vi "motor step1.vi"(8 "error in (no error)":errorcluster, 9 "direction":enum16{"counter-clockwise", "clockwise"}(ring), 10 "steps":i32=1, 11 "Handle In":i32) -> (0 "error out":errorcluster, 2 "steps performed":i32, 3 "Handle Out":i32)   [LabVIEW 2013]
uses:
  motor constants.ctl
  motor global state actions.ctl
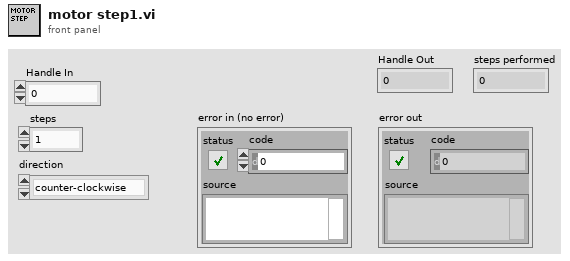
[diagram p1: front panel]
types:
  T1 = typedef "motor global state actions.ctl" = enum16{"set value", "get value", "set angle", "set initialized", "set complete", "set handle", "get handle"}
  T2 = typedef "motor constants.ctl" = u16
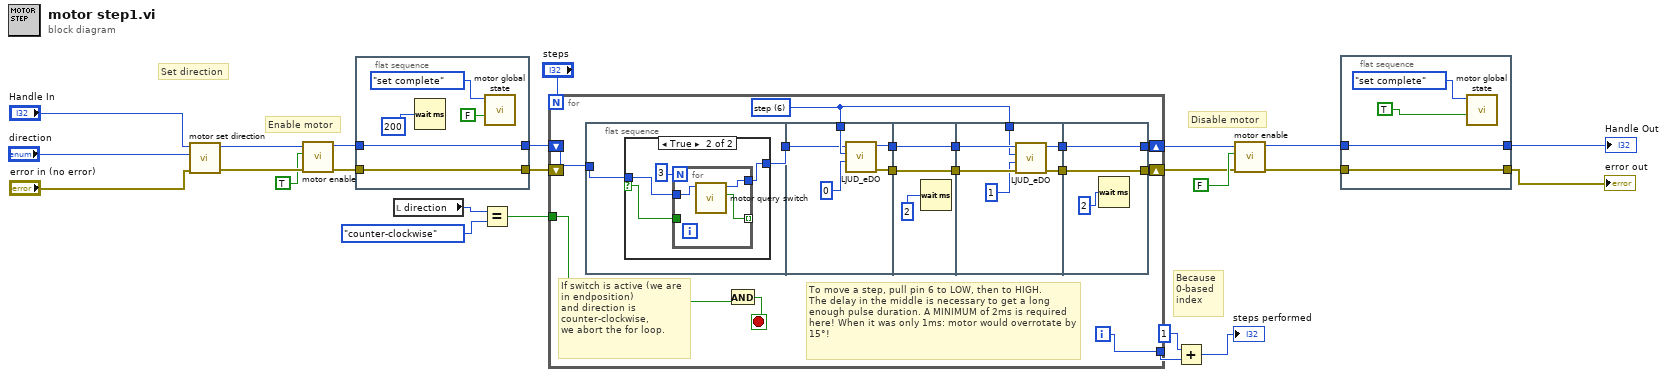
[diagram p0: block diagram]
diagram:
  # "Because \n0-based \nindex"
  # "Disable motor"
  # "Enable motor"
  # "Set direction"
  n1 = call "motor set direction.vi"("error in (no error)"="error in (no error)", "direction"="direction", "Handle In"="Handle In") -> ("error out"=w11:errorcluster, "Handle Out"=w10:i32)  [unwired: 7 in]
  n2 = call "motor enable.vi"("error in (no error)"=w11, "enable"=TRUE, "Handle In"=w10) -> ("error out"=w13:errorcluster, "Handle Out"=w12:i32)  [unwired: 7 in]
  n3 = flat-sequence {
    tunnel: w12 -> [w28]
    tunnel: w13 -> [w29]
    tunnel: [w29] -> w20
    tunnel: [w28] -> w19
    frame #0 {
      n4 = Wait (ms)(milliseconds to wait=200) -> ()  [unwired: 1 out]
      n5 = call "motor global state.vi"("completed"=FALSE, "action"=motor_global_state_actions."set complete" ("Motor FGV actions")) -> ()  [unwired: 8 in, 2 out]
    }
  }
  n6 = local read "direction"() -> (w23:enum16{"counter-clockwise", "clockwise"})
  n7 = Equal?(x=w23, y=enum16{"counter-clockwise", "clockwise"}."counter-clockwise" ("direction")) -> (x = y?=w21:bool)
  n8 = for {
    N: "steps" -> [_]
    tunnel: w21 -> [w32]
    tunnel: [w34] -> w3
    shift-right: [w42] -> w6
    shift-left: w19 -> [w30]
    shift-right: [w43] -> w7
    shift-left: w20 -> [_]
    i -> [w34]
    stop <- w33 stop-if-true
    w36 = T2 6 items=["enable"=4, "direction"=5, "step"=6, "end switch"=7] ("motor pin settings")
    # "To move a step, pull pin 6 to LOW, then to HIGH.\nThe delay in the middle is necessary to get a long enough pulse duration. A MINIMUM of 2ms is required here! When it was only 1ms: motor would overrotate by 15°!"
    # "If switch is active (we are in endposition)\nand direction is counter-clockwise,\nwe abort the for loop."
    n9 = flat-sequence {
      tunnel: w30 -> [w44]
      tunnel: [w45] -> w31
      tunnel: w36 -> [w57]
      tunnel: [w54] -> w38
      tunnel: [w55] -> w35
      tunnel: w31 -> [w53]
      tunnel: [w60] -> w39
      tunnel: w38 -> [w59]
      tunnel: [w59] -> w37
      tunnel: w35 -> [w60]
      tunnel: w39 -> [w66]
      tunnel: [w63] -> w41
      tunnel: w37 -> [w65]
      tunnel: [w64] -> w40
      tunnel: w36 -> [w61]
      tunnel: [w69] -> w43
      tunnel: w41 -> [w69]
      tunnel: [w68] -> w42
      tunnel: w40 -> [w68]
      frame #0 {
        n10 = case shown="True" {
          selector: _ -> [_ w46]
          tunnel: [_ w49] -> w45
          tunnel: w44 -> [_ w48]
          frame False {
          }
          frame True {
            n11 = for {
              N: 3 -> [_]
              tunnel: [w52] -> w49
              tunnel: w48 -> [w51]
              tunnel: w46 -> [_]
              tunnel: [w50] -> _ mode=indexing
              n12 = call "motor query switch.vi"("Handle In"=w51) -> ("switch state"=w50:bool, "Handle Out"=w52:i32)  [unwired: 8 in, 1 out]
            }
          }
        }
      }
      frame #1 {
        n13 = call <vilib>:"LJUD_eDO.vi"("State"=0, "Channel"=w57, "Handle In"=w53) -> ("error out"=w55:errorcluster, "Handle Out"=w54:i32)  [unwired: 7 in]
      }
      frame #2 {
        n14 = Wait (ms)(milliseconds to wait=2) -> ()  [unwired: 1 out]
      }
      frame #3 {
        n15 = call <vilib>:"LJUD_eDO.vi"("error in"=w66, "State"=1, "Channel"=w61, "Handle In"=w65) -> ("error out"=w63:errorcluster, "Handle Out"=w64:i32)  [unwired: 6 in]
      }
      frame #4 {
        n16 = Wait (ms)(milliseconds to wait=2) -> ()  [unwired: 1 out]
      }
    }
    n17 = And(y=w32) -> (x .and. y?=w33:bool)  [unwired: 1 in]
  }
  n18 = Add(x=1, y=w3) -> (x+y=→"steps performed":i32)
  n19 = call "motor enable.vi"("error in (no error)"=w7, "enable"=FALSE, "Handle In"=w6) -> ("error out"=w5:errorcluster, "Handle Out"=w4:i32)  [unwired: 7 in]
  n20 = flat-sequence {
    tunnel: w4 -> [w72]
    tunnel: w5 -> [w73]
    tunnel: [w73] -> w18
    tunnel: [w72] -> w17
    frame #0 {
      n21 = call "motor global state.vi"("completed"=TRUE, "action"=motor_global_state_actions."set complete" ("Motor FGV actions")) -> ()  [unwired: 8 in, 2 out]
    }
  }
  "Handle Out" <- w17
  "error out" <- w18
